vi "ClassPanel.vi"(8 "error in (no error)":errorcluster caption="entrée d'erreur (pas d'erreur)", 11 "ThorPM100A.lvclass":refnum<class "ThorPM100A.lvclass">) -> (0 "error out":errorcluster caption="sortie d'erreur", 3 "ThorPM100A.lvclass Out":refnum<class "ThorPM100A.lvclass">)   [LabVIEW 2019, in "ThorPM100A.lvclass"]
uses:
  ThorPM100A.lvclass
  C:/Programmes Labview/LabscanV1A/DevicesClass/BaseDevice/BaseDevice.lvclass
  ThorPM100A.lvclass/ThorPM100A.ctl
  BaseDevice/ClassQueueMess.ctl
  BaseDevice/BaseDevice.lvclass/BaseDevice.ctl
  BaseDevice/Accessor/GetBaseDataPath.vi
  BaseDevice/Accessor/GetClassEvent.vi
  <vilib>/Utility/error.llb/Error Cluster From Error Code.vi
  <vilib>/ErrorRing/Error Ring.xnode
panel:
  in  "TrigSourceRef":refnum<vi>
  out "ClearG":refnum<vi>
  in  "Clear":bool caption="MiseAJour"
  out "BaseDataPath":path
  out "VisaRes":refnum<visa-resource-name>
  out "AvgRef":refnum<vi>
  out "ViRef":refnum<vi>
  out "GraphRef":refnum<vi>
  out "DataRef":refnum<vi>
  out "GraphAct":bool
  in  "Graph":bool
  out "StartTime":dbl
  in  "PwIdx":i32
  out "PowerData":dbl[](array[numeric])
  out "Refresh count":u32=1 caption="Panel Refresh (s-1)" min=1 max=5 step=1
  in  "Panel Refresh":dbl=1.0 caption="Panel Refresh (s)" min=0.2 max=1000.0 step=0.2
  in  "Record":bool
  in  "Zero":bool
  in  "Conn/Dis":bool
  in  "Average":i16=60 caption="Average Cnt"
  in  "Attenuation":dbl=60.0 caption="Atten.(dB)" format="%^#.2e"
  in  "Range":dbl=60.0 caption="Range (W)" format="%^#.2e"
  in  "Autorange":bool
  in  "MainProgQ":refnum<queue>
  in  "MainProgQEvent":refnum<user-event>
  in  "Acq":bool
  in  "Stop":bool
  in  "Wavelength":dbl caption="Lambda(nm)" format="%.1f"
  in  "MiseAJour":bool
  out "Power":dbl=60.0 caption="Power (W)" min=0.1 step=0.1 format="%^#.3e"
  out "Init Program":bool
  # "PM100A PowerMeter"
  # "this MUST labeled with class name"
  # "this MUST be present and labeled \"Stop\" and \"Acq\""
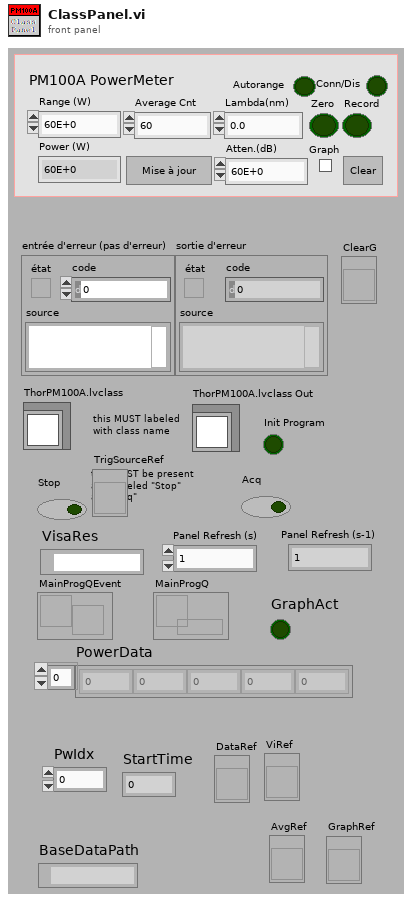
[diagram p1: front panel]
types:
  T1 = enum32{"Invalid", "Standard", "Closed", "Hidden", "Minimized", "Maximized"}
  T2 = cluster{"Max Val":dbl, "Curr.Val":dbl, "Meas.Avg":dbl, "Range":dbl}
  T3 = typedef "ClassQueueMess.ctl" = u16
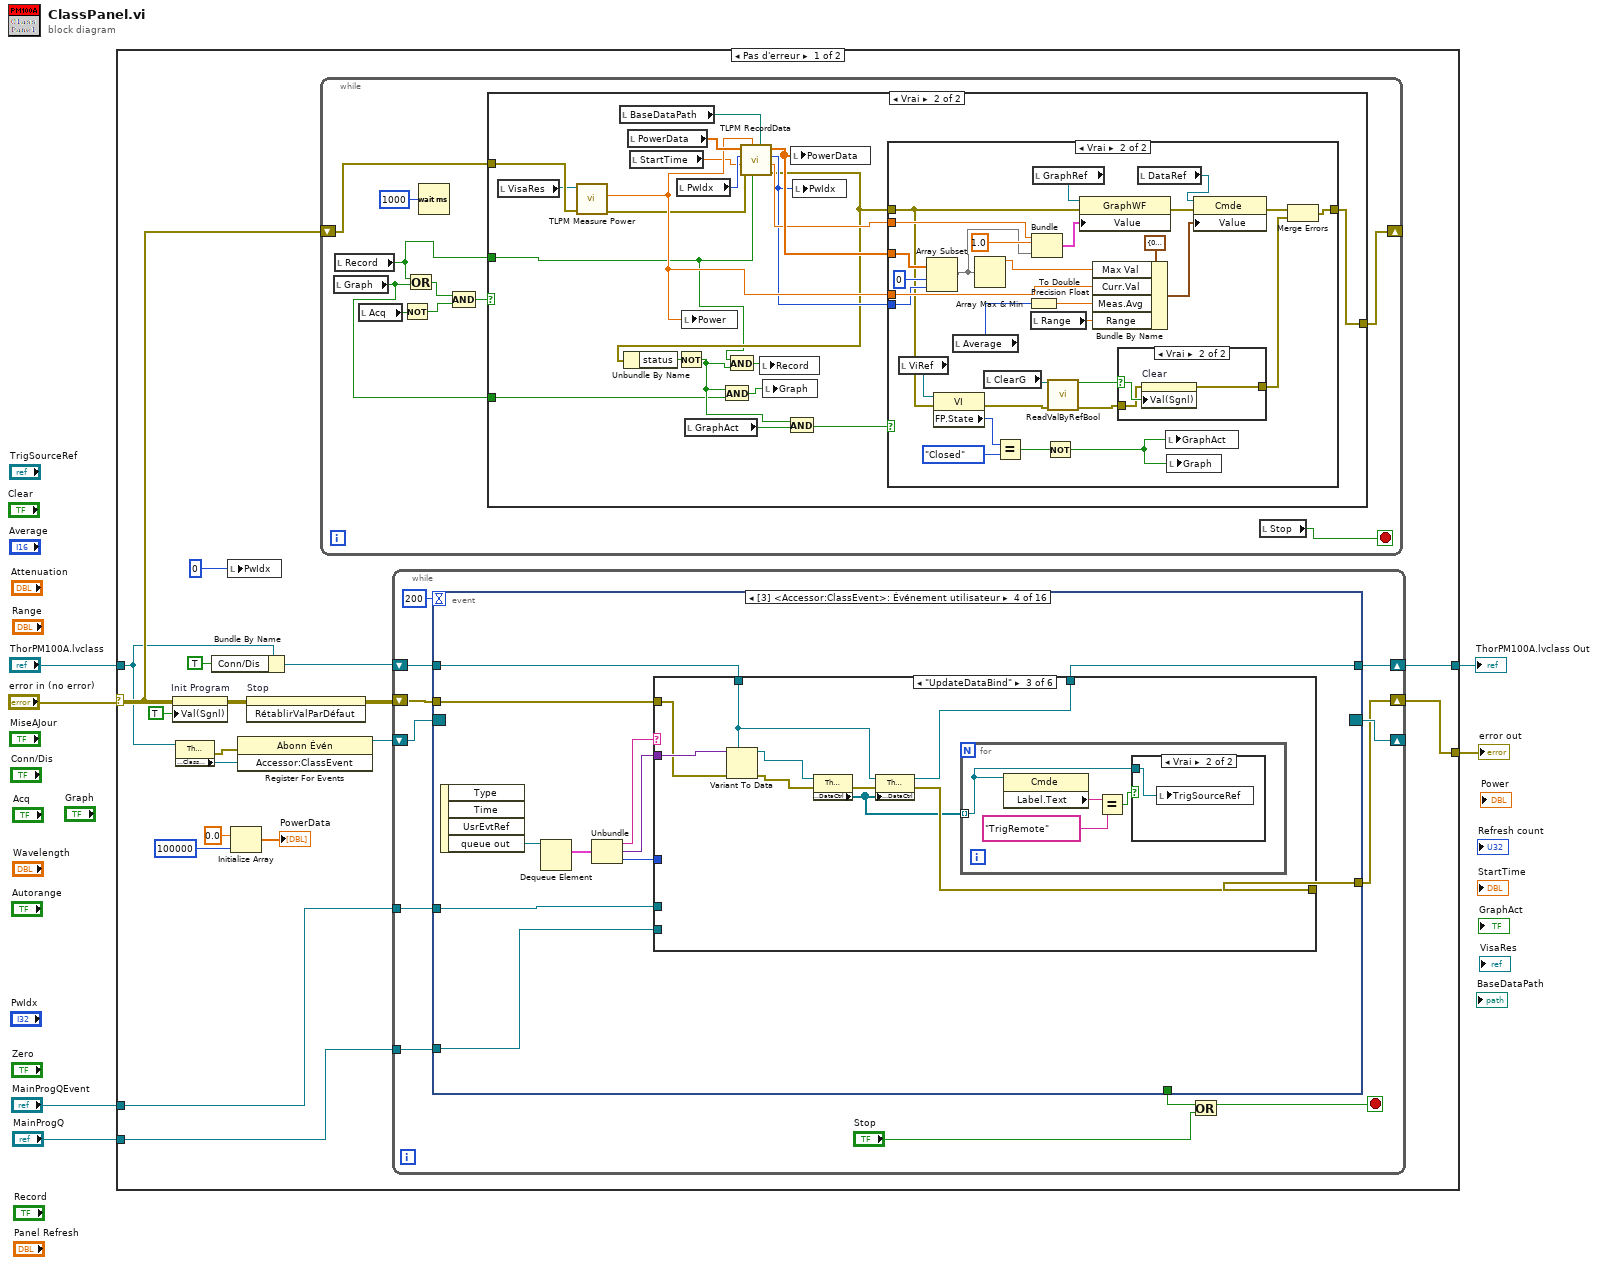
[diagram p0: block diagram]
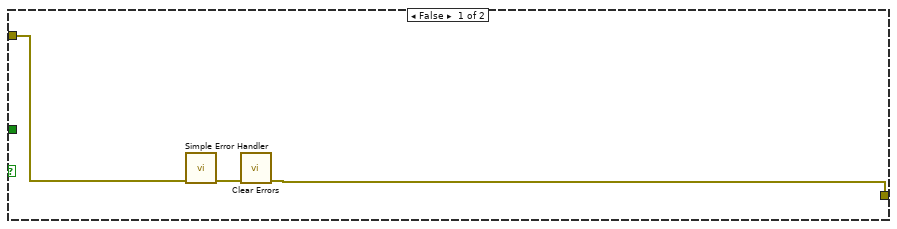
[diagram p2: hidden frame]
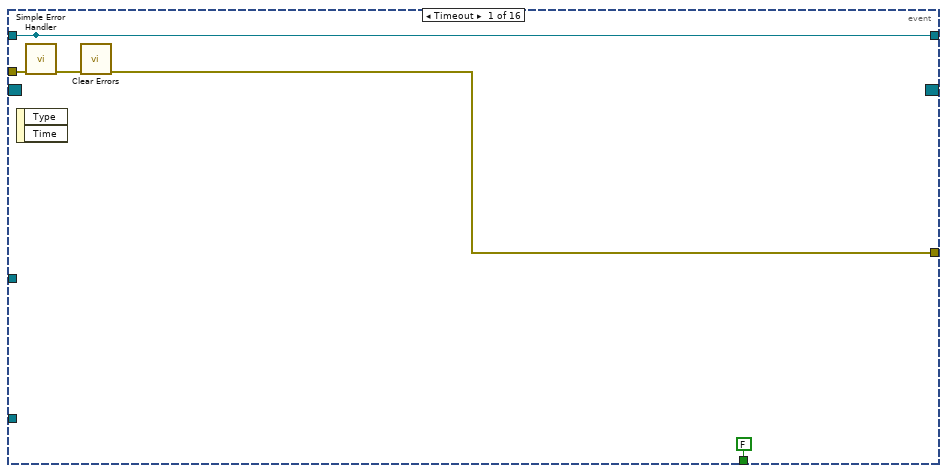
[diagram p5: hidden frame]
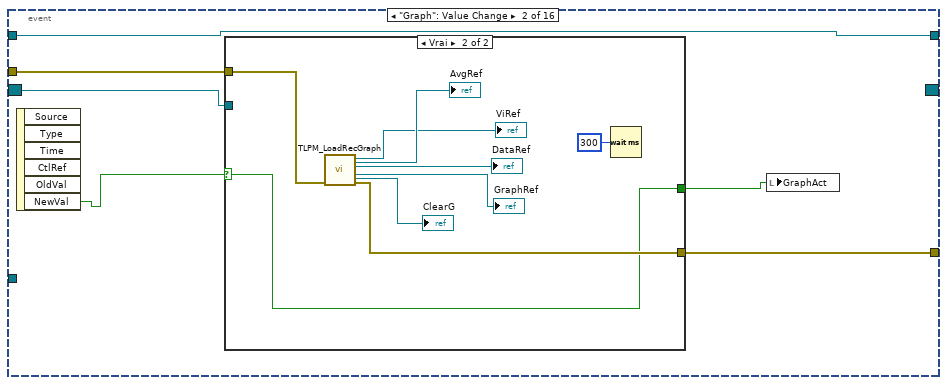
[diagram p6: hidden frame]
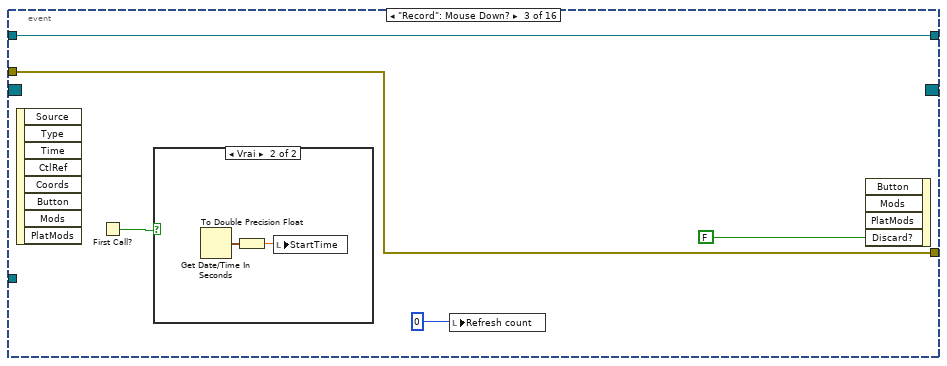
[diagram p8: hidden frame]
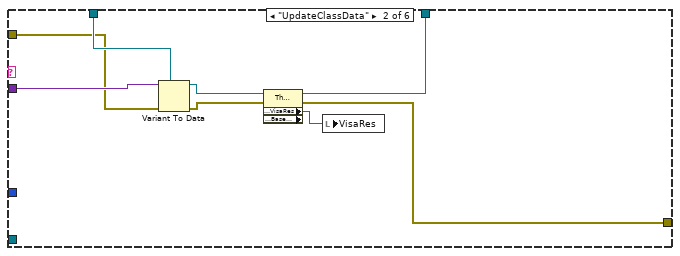
[diagram p11: hidden frame]
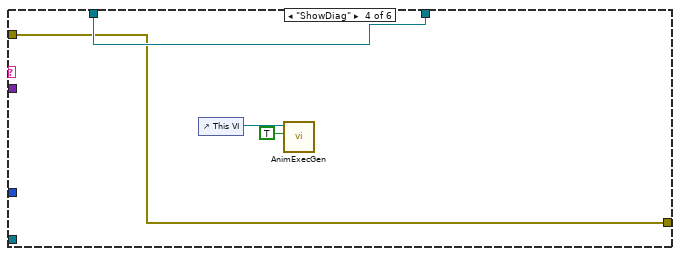
[diagram p13: hidden frame]
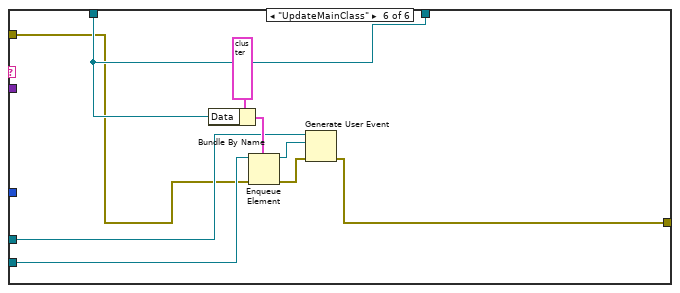
[diagram p15: hidden frame]
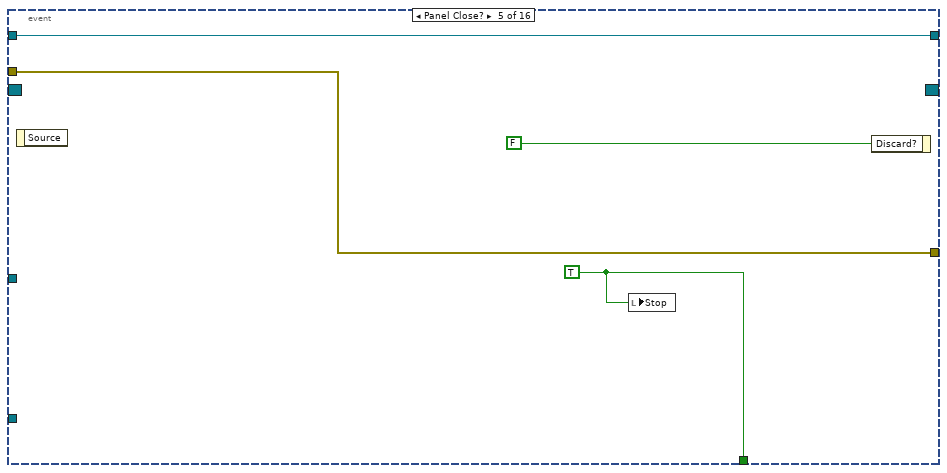
[diagram p16: hidden frame]
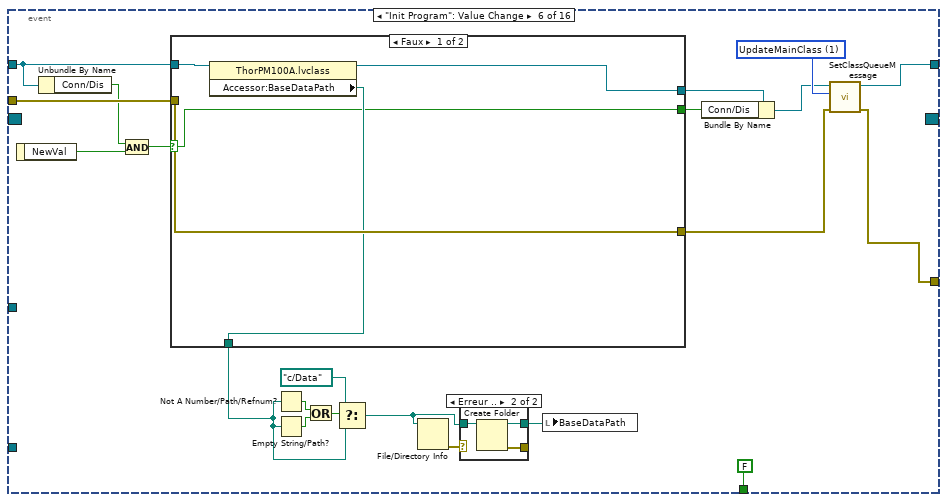
[diagram p17: hidden frame]
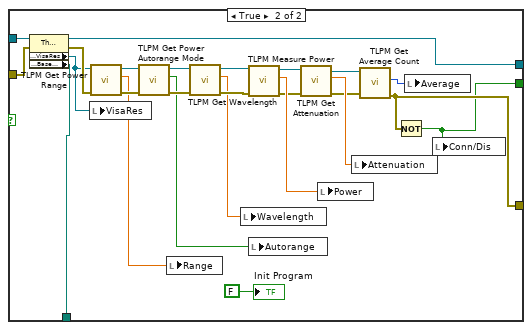
[diagram p19: hidden frame]
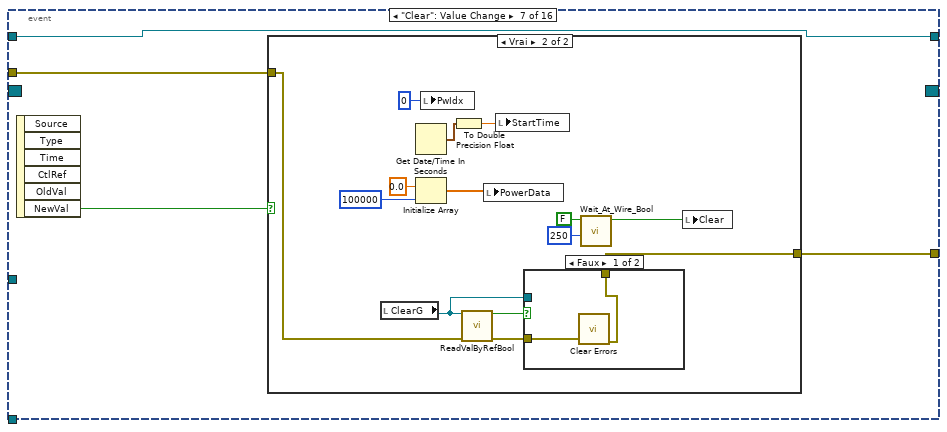
[diagram p20: hidden frame]
diagram:
  n1 = case shown="Pas d'erreur" "error in (no error)" {
    selector: "error in (no error)" -> [w10 w449]
    tunnel: [w24 w449] -> w5
    tunnel: "ThorPM100A.lvclass" -> [w9 w448]
    tunnel: [w22 w448] -> w3
    tunnel: "MainProgQEvent" -> [w16 _]
    tunnel: "MainProgQ" -> [w15 _]
    frame No Error {
      n2 = property on="Init Program" class="Bool (strict)"(error in=w10, "Val(Sgnl)"=TRUE ("Valeur (Signalisation)")) -> (error out=w21:errorcluster)  [unwired: 1 in, 1 out]
      n3 = property class="ThorPM100A.lvclass"(reference=w9) -> (error out=w19:errorcluster, "Accessor:ClassEvent"=w18:refnum<user-event>)  [unwired: 1 in, 1 out]
      n4 = Bundle By Name(cluster=w9, "Conn/Dis"=TRUE) -> (w7:refnum<class "ThorPM100A.lvclass">)
      n5 = local write "PwIdx"(u32 0 ("Power index")) -> ()
      n6 = Initialize Array(0.0 ("élément"), 100000 ("taille de la dimension")) -> (→"PowerData":dbl[])
      n7 = register-events(error in=w19, w18) -> (reference out=w17:refnum<event-registration>)  [unwired: 1 in, 1 out]
      n8 = invoke on="Stop" class="Bool (strict)" method="RétablirValParDéfaut"(error in=w21) -> (error out=w20:errorcluster)  [unwired: 2 in, 2 out]
      n9 = while {
        shift-right: [w28] -> _
        shift-left: w10 -> [w29]
        stop <- w32 stop-if-true
        n10 = local read "Graph"() -> (w25:bool)
        n11 = local read "Record"() -> (w26:bool)
        n12 = local read "Acq"() -> (w33:bool)
        n13 = Not(x=w33) -> (.not. x?=w34:bool)
        n14 = Or(x=w26, y=w25) -> (x .or. y?=w27:bool)
        n15 = Wait (ms)(milliseconds to wait=u32 1000 ("attente (ms)")) -> ()  [unwired: 1 out]
        n16 = Compound Arithmetic op=AND ("Opérateur arithmétique")(w27, w34) -> (w30:bool)
        n17 = case shown="Vrai" w30 {
          tunnel: [w35 w58] -> w28
          tunnel: w29 -> [w36 w49]
          tunnel: w26 -> [_ w41]
          tunnel: w25 -> [_ w38]
          frame False {
            n18 = call <vilib>:"Simple Error Handler.vi"("error in (no error)"=w36) -> ("error out"=w37:errorcluster)  [unwired: 4 in, 4 out]
            n19 = call <vilib>:"Clear Errors.vi"("error in (no error)"=w37) -> ("error out"=w35:errorcluster)  [unwired: 5 in, 1 out]
          }
          frame True {
            n20 = local read "VisaRes"() -> (w48:refnum<visa-resource-name>)
            n21 = call <instrlib>:"TLPM Measure Power.vi"("error in (no error)"=w49, "instrument handle"=w48) -> ("error out"=w45:errorcluster, "Power"=w53:dbl)  [unwired: 7 in, 1 out]
            n22 = local read "BaseDataPath"() -> (w46:path)
            n23 = local read "PowerData"() -> (w55:dbl[])
            n24 = local read "StartTime"() -> (w51:dbl)
            n25 = local read "PwIdx"() -> (w52:i32)
            n26 = local write "Power"(w53) -> ()
            n27 = local read "GraphAct"() -> (w56:bool)
            n28 = call "TLPM RecordData.vi"("BaseDataPath"=w46, "Save"=w41, "Power In"=w53, "error in (no error)"=w45, "StartTimeIn"=w51, "PwIdxIn"=w52, "PowerDataIn"=w55) -> ("error out"=w44:errorcluster, "StartTime"=w50:dbl, "PwIdxOut"=w47:i32, "PowerData"=w54:dbl[])  [unwired: 1 in]
            n29 = Unbundle By Name(w44) -> ("status"=w57:bool)
            n30 = Not(x=w57) -> (.not. x?=w40:bool)
            n31 = And(x=w40, y=w38) -> (x .and. y?=w39:bool)
            n32 = And(x=w41, y=w40) -> (x .and. y?=w42:bool)
            n33 = local write "Record"(w42) -> ()
            n34 = local write "Graph"(w39) -> ()
            n35 = And(x=w40, y=w56) -> (x .and. y?=w43:bool)
            n36 = local write "PowerData"(w54) -> ()
            n37 = local write "PwIdx"(w47) -> ()
            n38 = case shown="Vrai" w43 {
              tunnel: [w59 w64] -> w58
              tunnel: w44 -> [w59 w62]
              tunnel: w53 -> [_ w85]
              tunnel: w50 -> [_ w84]
              tunnel: w54 -> [_ w71]
              tunnel: w47 -> [_ w69]
              frame False {
              }
              frame True {
                n39 = local read "ViRef"() -> (w67:refnum<vi>)
                n40 = Array Subset(array=w71, index=0 ("indice"), length=w69) -> (w68:dbl[])
                n41 = property class="VI"(reference=w67, error in=w62) -> (error out=w61:errorcluster, "FP.State"=w81:T1)  [unwired: 1 out]
                n42 = local read "Average"() -> (w74:i16)
                n43 = Array Max & Min(array=w68) -> (max value=w75:dbl)  [unwired: 3 out]
                n44 = local read "ClearG"() -> (w60:refnum<vi>)
                n45 = Equal?(x=w81, y=T1."Closed") -> (x = y?=w79:bool)
                n46 = To Double Precision Float(number=w74) -> (double precision float=w73:dbl)
                n47 = local read "Range"() -> (w88:dbl)
                n48 = Bundle("StartTime"=w84, 1.0, w68) -> (w83:cluster{"StartTime":dbl, dbl, dbl[]})  [unwired: 1 in]
                n49 = local read "GraphRef"() -> (w82:refnum<vi>)
                n50 = Not(x=w79) -> (.not. x?=w78:bool)
                n51 = call <userlib>:"ReadValByRefBool.vi"("Control Ref"=w60, "error in"=w61) -> ("Valeur"=w66:bool, "error out"=w65:errorcluster)  [unwired: 12 in]
                n52 = property class="GraphWF"(reference=w82, error in=w62, "Value"=w83) -> (error out=w87:errorcluster)  [unwired: 1 out]
                n53 = Bundle By Name(cluster=T2 {"Max Val"=0.0, "Curr.Val"=0.0, "Meas.Avg"=0.0, "Range"=0.0} ("Data"), "Max Val"=w75, "Curr.Val"=w85, "Meas.Avg"=w73, "Range"=w88) -> (w76:T2)
                n54 = case shown="Vrai" w66 {
                  selector: w66 -> [_ w93]
                  tunnel: w65 -> [w90 w92]
                  tunnel: [w90 w91] -> w63
                  frame False {
                  }
                  frame True {
                    n55 = property on="Clear" class="Bool (strict)"(error in=w92, "Val(Sgnl)"=w93) -> (error out=w91:errorcluster)  [unwired: 1 in, 1 out]
                  }
                }
                n56 = local read "DataRef"() -> (w77:refnum<vi>)
                n57 = local write "GraphAct"(w78) -> ()
                n58 = local write "Graph"(w78) -> ()
                n59 = property class="Cmde"(reference=w77, error in=w87, "Value"=w76) -> (error out=w86:errorcluster)  [unwired: 1 out]
                n60 = Merge Errors(w86, w63) -> (w64:errorcluster)
              }
            }
          }
        }
        n61 = local read "Stop"() -> (w32:bool)
      }
      n62 = while {
        shift-right: [w94] -> w24
        shift-left: w20 -> [w104]
        shift-right: [w101] -> w22
        shift-left: w7 -> [w103]
        shift-right: [w97] -> _
        shift-left: w17 -> [w98]
        tunnel: w16 -> [w96]
        tunnel: w15 -> [w95]
        stop <- w100 stop-if-true
        n63 = event shown="[3] <Accessor:ClassEvent>: Événement utilisateur" {
          selector: w98 -> [_ w113 _ _ _ _ _ _ _ _ _ _ _ _ _ _]
          dyn-events: [_ _ _ _ _ _ _ _ _ _ _ _ _ _ _ _] -> w97
          timeout: 200 -> [_ _ _ _ _ _ _ _ _ _ _ _ _ _ _ _]
          tunnel: w104 -> [w109 w115 w131 w144 w187 w209 w245 w274 w312 w339 w389 w399 w409 w419 w427 w446]
          tunnel: [w106 w114 w131 w138 w187 w190 w246 w273 w311 w334 w386 w394 w405 w415 w423 w443] -> w94
          tunnel: w103 -> [w107 w111 w130 w145 w186 w207 w247 w271 w314 w340 w390 w400 w410 w420 w428 w447]
          tunnel: [FALSE _ _ _ w185 FALSE _ FALSE _ _ _ _ _ _ _ _] -> w102
          tunnel: [w107 w111 w130 w137 w186 w189 w247 w270 w313 w337 w385 w396 w408 w418 w426 w442] -> w101
          tunnel: w96 -> [_ _ _ w136 _ _ _ _ _ _ _ _ _ _ _ _]
          tunnel: w95 -> [_ _ _ w135 _ _ _ _ _ _ _ _ _ _ _ _]
          tunnel: [w107 _ _ _ _ _ _ _ _ _ _ _ _ _ _ _] -> _
          event Timeout {
            n64 = event-data() -> ()  [unwired: 1 in, 2 out]
            n65 = call <vilib>:"Simple Error Handler.vi"("error in (no error)"=w109) -> ("error out"=w108:errorcluster)  [unwired: 4 in, 4 out]
            n66 = call <vilib>:"Clear Errors.vi"("error in (no error)"=w108) -> ("error out"=w106:errorcluster)  [unwired: 5 in, 1 out]
          }
          event "Graph": Value Change {
            n67 = event-data() -> ("NewVal"=w116:bool)  [unwired: 1 in, 5 out]
            n68 = case shown="Vrai" w116 {
              selector: w116 -> [w117 w120]
              tunnel: w115 -> [w118 w127]
              tunnel: [w118 w122] -> w114
              tunnel: w113 -> [_ _]
              tunnel: [w117 w120] -> w112
              frame False {
              }
              frame True {
                n69 = call <instrlib>:"TLPM_LoadRecGraph.vi"("ErrIn(No Err)"=w127) -> ("ErrOut"=w122:errorcluster, "Graph"=→"GraphRef":refnum<vi>, "Data"=→"DataRef":refnum<vi>, "ViRef"=→"ViRef":refnum<vi>, "Clear"=→"ClearG":refnum<vi>, "Avg ref"=→"AvgRef":refnum<vi>)  [unwired: 5 in]
                n70 = Wait (ms)(milliseconds to wait=u32 300 ("attente (ms)")) -> ()  [unwired: 1 out]
              }
            }
            n71 = local write "GraphAct"(w112) -> ()
          }
          event "Record": Mouse Down? {
            n72 = event-data() -> ()  [unwired: 1 in, 8 out]
            n73 = First Call?() -> (First Call?: T/F=w129:bool)
            n74 = case shown="Vrai" w129 {
              frame False {
              }
              frame True {
                n75 = Get Date/Time In Seconds() -> (seconds since 1Jan1904=w134:timestamp)
                n76 = To Double Precision Float(number=w134) -> (double precision float=w133:dbl)
                n77 = local write "StartTime"(w133) -> ()
              }
            }
            n78 = local write "Refresh count"(u32 0 ("Refresh count")) -> ()
            n79 = event-data("Discard?"=FALSE ("Rejeter ?")) -> ()  [unwired: 4 in, 1 out]
          }
          event User Event {
            n80 = event-data() -> ("queue out"=w142:refnum<queue>)  [unwired: 1 in, 3 out]
            n81 = Dequeue Element(queue=w142) -> (element=w143:cluster{"Message":string, "Data":variant, i32})  [unwired: 2 in, 3 out]
            n82 = Unbundle(w143) -> ("Message"=w141:string, "Data"=w140:variant, w139:i32)
            n83 = case shown="\"UpdateDataBind\"" w141 {
              tunnel: w144 -> [w147 w151 w163 w170 w174 w177]
              tunnel: w140 -> [_ w155 w164 _ _ _]
              tunnel: w145 -> [w146 w154 w159 w171 w175 w180]
              tunnel: [w146 w152 w156 w171 w175 w180] -> w137
              tunnel: [w147 w149 w158 w170 w174 w176] -> w138
              tunnel: w139 -> [_ _ _ _ _ _]
              tunnel: w136 -> [_ _ _ _ _ w179]
              tunnel: w135 -> [_ _ _ _ _ w178]
              frame Default {
              }
              frame "UpdateClassData" {
                n84 = Variant To Data(error in=w151, type=w154, Variant=w155) -> (data=w153:refnum<class "ThorPM100A.lvclass">, error out=w150:errorcluster)
                n85 = property class="ThorPM100A.lvclass" props=["Accessor:VisaRes", "Accessor:BaseDataPath"](reference=w153, error in=w150) -> (reference out=w152:refnum<class "ThorPM100A.lvclass">, error out=w149:errorcluster, "Accessor:VisaRes"=w148:refnum<visa-resource-name>)  [unwired: 1 out]
                n86 = local write "VisaRes"(w148) -> ()
              }
              frame "UpdateDataBind" {
                n87 = Variant To Data(error in=w163, type=w159, Variant=w164) -> (data=w160:refnum<class "ThorPM100A.lvclass">, error out=w161:errorcluster)
                n88 = property class="ThorPM100A.lvclass"(reference=w160, error in=w161) -> (error out=w162:errorcluster, "Accessor:DataCtrl"=w157:refnum<vi>[])  [unwired: 1 out]
                n89 = property class="ThorPM100A.lvclass"(reference=w159, error in=w162, "Accessor:DataCtrl"=w157) -> (reference out=w156:refnum<class "ThorPM100A.lvclass">, error out=w158:errorcluster)
                n90 = for {
                  tunnel: w157 -> [w165] mode=indexing
                  n91 = property class="Cmde"(reference=w165) -> ("Label.Text"=w168:string)  [unwired: 1 in, 2 out]
                  n92 = Equal?(x=w168, y="TrigRemote") -> (x = y?=w166:bool)
                  n93 = case shown="Vrai" w166 {
                    tunnel: w165 -> [_ w169]
                    frame False {
                    }
                    frame True {
                      n94 = local write "TrigSourceRef"(w169) -> ()
                    }
                  }
                }
              }
              frame "ShowDiag" {
                n95 = control-ref of="This VI"() -> (w173:refnum<vi>)
                n96 = call <userlib>:"AnimExecGen.vi"("Animer l'exécution ?"=TRUE, "ViRef"=w173) -> ()  [unwired: 9 in, 1 out]
              }
              frame "MeasDone" {
              }
              frame "UpdateMainClass" {
                n97 = Bundle By Name(cluster=cluster{"Message":string, "Data":variant, i32} {"Message"="", "Data"=variant, 0} ("élément"), "Data"=w180) -> (w181:cluster{"Message":string, "Data":variant, i32})
                n98 = Enqueue Element(queue=w178, element=w181, error in (no error)=w177) -> (queue out=w184:refnum<queue>, error out=w183:errorcluster)  [unwired: 1 in, 1 out]
                n99 = Generate User Event(user event=w179, event data cluster=w184, error in=w183) -> (error out=w176:errorcluster)  [unwired: 1 in, 1 out]
              }
            }
          }
          event Panel Close? {
            w185 = TRUE
            n100 = event-data() -> ()  [unwired: 1 in, 1 out]
            n101 = local write "Stop"(w185) -> ()
            n102 = event-data("Discard?"=FALSE ("Rejeter ?")) -> ()  [unwired: 1 in, 1 out]
          }
          event "Init Program": Value Change {
            w193 = T3 1 items=["UpdateClassData", "UpdateMainClass", "UpdateDataBind", "ReInitDevice", "Custom", "ClosePan"] ("Menu déroulant")
            n103 = event-data() -> ("NewVal"=w204:bool)  [unwired: 1 in]
            n104 = Unbundle By Name(w207) -> ("Conn/Dis"=w205:bool)
            n105 = And(x=w205, y=w204) -> (x .and. y?=w206:bool)
            n106 = case shown="Faux" w206 {
              selector: w206 -> [w215 _]
              tunnel: w209 -> [w219 w241]
              tunnel: [w219 w225] -> w191
              tunnel: w207 -> [w218 w243]
              tunnel: [w217 w242] -> w195
              tunnel: [w216 w221] -> w196
              tunnel: [w215 w220] -> w194
              frame False {
                n107 = property class="ThorPM100A.lvclass"(reference=w218) -> (reference out=w217:refnum<class "ThorPM100A.lvclass">, "Accessor:BaseDataPath"=w216:path)  [unwired: 1 in, 1 out]
              }
              frame True {
                n108 = property class="ThorPM100A.lvclass"(reference=w243, error in=w241) -> (reference out=w242:refnum<class "ThorPM100A.lvclass">, error out=w240:errorcluster, "Accessor:VisaRes"=w222:refnum<visa-resource-name>, "Accessor:BaseDataPath"=w221:path)
                n109 = local write "VisaRes"(w222) -> ()
                n110 = call <instrlib>:"TLPM Get Power Range.vi"("error in (no error)"=w240, "instrument handle"=w222) -> ("error out"=w238:errorcluster, "Power Value"=w230:dbl, "instrument handle out"=w239:refnum<visa-resource-name>)  [unwired: 7 in]
                n111 = call <instrlib>:"TLPM Get Power Autorange Mode.vi"("error in (no error)"=w238, "instrument handle"=w239) -> ("error out"=w236:errorcluster, "Power Autorange Mode"=w235:bool, "instrument handle out"=w237:refnum<visa-resource-name>)  [unwired: 7 in]
                n112 = local write "Range"(w230) -> ()
                n113 = call <instrlib>:"TLPM Get Wavelength.vi"("error in (no error)"=w236, "instrument handle"=w237) -> ("error out"=w233:errorcluster, "Wavelength"=w232:dbl, "instrument handle out"=w234:refnum<visa-resource-name>)  [unwired: 7 in]
                n114 = local write "Wavelength"(w232) -> ()
                n115 = call <instrlib>:"TLPM Measure Power.vi"("error in (no error)"=w233, "instrument handle"=w234) -> ("error out"=w228:errorcluster, "Power"=w231:dbl, "instrument handle out"=w229:refnum<visa-resource-name>)  [unwired: 7 in]
                n116 = local write "Autorange"(w235) -> ()
                n117 = call <instrlib>:"TLPM Get Attenuation.vi"("error in (no error)"=w228, "instrument handle"=w229) -> ("error out"=w226:errorcluster, "Attenuation"=w227:dbl, "instrument handle out"=w224:refnum<visa-resource-name>)  [unwired: 7 in]
                n118 = local write "Power"(w231) -> ()
                n119 = local write "Attenuation"(w227) -> ()
                n120 = call <instrlib>:"TLPM Get Average Count.vi"("error in (no error)"=w226, "instrument handle"=w224) -> ("error out"=w225:errorcluster, "Average Count"=w223:i16)  [unwired: 7 in, 1 out]
                n121 = Not(x=w225) -> (.not. x?=w220:bool)
                n122 = local write "Average"(w223) -> ()
                n123 = local write "Conn/Dis"(w220) -> ()
                "Init Program" <- FALSE
              }
            }
            n124 = Not A Number/Path/Refnum?(number/path/refnum=w196) -> (NaN/Path/Refnum?=w202:bool)
            n125 = Empty String/Path?(string/path=w196) -> (empty?=w201:bool)
            n126 = Or(x=w202, y=w201) -> (x .or. y?=w200:bool)
            n127 = Select(t=path "c:/Data" ("cas vrai"), s=w200, f=w196) -> (s? t:f=w199:path)
            n128 = File/Directory Info(path=w199) -> (error out=w203:errorcluster)  [unwired: 1 in, 6 out]
            n129 = case shown="Erreur .." w203 {
              selector: w203 -> [w211 _]
              tunnel: w199 -> [w210 w214]
              tunnel: [w211 w213] -> _
              tunnel: [w210 w212] -> w198
              frame No Error {
              }
              frame Error {
                n130 = Create Folder(path (use dialog)=w214) -> (created path=w212:path, error out=w213:errorcluster)  [unwired: 2 in, 1 out]
              }
            }
            n131 = local write "BaseDataPath"(w198) -> ()
            n132 = Bundle By Name(cluster=w195, "Conn/Dis"=w194) -> (w192:refnum<class "ThorPM100A.lvclass">)
            n133 = call-dynamic "SetClassQueueMessage.vi"("ErrorIn(No Error)"=w191, "Menu déroulant"=w193, "DefaultDev.lvclass"=w192) -> ("sortie d'erreur"=w190:errorcluster, "DefaultDev.lvclass Out"=w189:refnum<class "ThorPM100A.lvclass">)  [unwired: 7 in]
          }
          event "Clear": Value Change {
            n134 = event-data() -> ("NewVal"=w248:bool)  [unwired: 1 in, 5 out]
            n135 = case shown="Vrai" w248 {
              tunnel: [w249 w251] -> w246
              tunnel: w245 -> [w249 w250]
              frame False {
              }
              frame True {
                n136 = local read "ClearG"() -> (w252:refnum<vi>)
                n137 = Get Date/Time In Seconds() -> (seconds since 1Jan1904=w256:timestamp)
                n138 = Initialize Array(0.0 ("élément"), 100000 ("taille de la dimension")) -> (w257:dbl[])
                n139 = local write "PwIdx"(0 ("PwIdx")) -> ()
                n140 = To Double Precision Float(number=w256) -> (double precision float=w255:dbl)
                n141 = call <userlib>:"ReadValByRefBool.vi"("Control Ref"=w252, "error in"=w250) -> ("Valeur"=w254:bool, "error out"=w253:errorcluster)  [unwired: 12 in]
                n142 = local write "PowerData"(w257) -> ()
                n143 = local write "StartTime"(w255) -> ()
                n144 = case shown="Faux" w254 {
                  tunnel: w253 -> [w265 w267]
                  tunnel: w252 -> [_ w269]
                  tunnel: [w264 w266] -> w251
                  frame False {
                    n145 = call <vilib>:"Clear Errors.vi"("error in (no error)"=w265) -> ("error out"=w264:errorcluster)  [unwired: 5 in, 1 out]
                  }
                  frame True {
                    n146 = call <userlib>:"WritebyWeakRefBool.vi"("error in"=w267, "Valeur"=FALSE, "Control Ref"=w269) -> ("error out"=w266:errorcluster)  [unwired: 8 in]
                  }
                }
                n147 = call <userlib>:"Wait_At_Wire_Bool.vi"("Wait (ms)"=u32 250, "error in (no error)"=FALSE) -> ("error out"=w263:bool)  [unwired: 7 in, 2 out]
                n148 = local write "Clear"(w263) -> ()
              }
            }
          }
          event "MiseAJour": Value Change {
            n149 = event-data() -> ("NewVal"=w275:bool)  [unwired: 1 in]
            n150 = case shown="Vrai" w275 {
              tunnel: w274 -> [w277 w302]
              tunnel: [w277 w280] -> w273
              tunnel: w271 -> [w276 w304]
              tunnel: [w276 w303] -> w270
              frame False {
              }
              frame True {
                n151 = property class="ThorPM100A.lvclass"(reference=w304, error in=w302) -> (reference out=w303:refnum<class "ThorPM100A.lvclass">, error out=w301:errorcluster, "Accessor:VisaRes"=w286:refnum<visa-resource-name>)
                n152 = call <instrlib>:"TLPM Get Power Range.vi"("error in (no error)"=w301, "instrument handle"=w286) -> ("error out"=w299:errorcluster, "Power Value"=w293:dbl, "instrument handle out"=w300:refnum<visa-resource-name>)  [unwired: 7 in]
                n153 = call <instrlib>:"TLPM Get Power Autorange Mode.vi"("error in (no error)"=w299, "instrument handle"=w300) -> ("error out"=w288:errorcluster, "Power Autorange Mode"=w298:bool, "instrument handle out"=w287:refnum<visa-resource-name>)  [unwired: 7 in]
                n154 = local write "Range"(w293) -> ()
                n155 = Wait (ms)(milliseconds to wait=u32 300 ("attente (ms)")) -> (millisecond timer value=w292:u32)
                n156 = call <instrlib>:"TLPM Get Wavelength.vi"("error in (no error)"=w288, "instrument handle"=w287) -> ()  [unwired: 7 in, 3 out]
                n157 = call <instrlib>:"TLPM Get Wavelength.vi"("error in (no error)"=w288, "instrument handle"=w287) -> ("error out"=w296:errorcluster, "Wavelength"=w295:dbl, "instrument handle out"=w297:refnum<visa-resource-name>)  [unwired: 7 in]
                n158 = flat-sequence {
                  tunnel: w292 -> [_]
                  frame #0 {
                    n159 = local write "MiseAJour"(FALSE ("MiseAJour")) -> ()
                  }
                }
                n160 = local write "Wavelength"(w295) -> ()
                n161 = call <instrlib>:"TLPM Measure Power.vi"("error in (no error)"=w296, "instrument handle"=w297) -> ("error out"=w290:errorcluster, "Power"=w294:dbl, "instrument handle out"=w289:refnum<visa-resource-name>)  [unwired: 7 in]
                n162 = local write "Autorange"(w298) -> ()
                n163 = local read "TrigSourceRef"() -> (w279:refnum<vi>)
                n164 = call <instrlib>:"TLPM Get Attenuation.vi"("error in (no error)"=w290, "instrument handle"=w289) -> ("error out"=w283:errorcluster, "Attenuation"=w285:dbl, "instrument handle out"=w282:refnum<visa-resource-name>)  [unwired: 7 in]
                n165 = local write "Attenuation"(w285) -> ()
                n166 = local write "Power"(w294) -> ()
                n167 = call <instrlib>:"TLPM Get Average Count.vi"("error in (no error)"=w283, "instrument handle"=w282) -> ("error out"=w281:errorcluster, "Average Count"=w284:i16)  [unwired: 7 in, 1 out]
                n168 = local write "Average"(w284) -> ()
                n169 = Not A Number/Path/Refnum?(number/path/refnum=w279) -> (NaN/Path/Refnum?=w278:bool)
                n170 = case shown="Faux" w278 {
                  tunnel: w281 -> [w308 w309]
                  tunnel: [w307 w309] -> w280
                  tunnel: w279 -> [w306 _]
                  frame False {
                    n171 = call <userlib>:"WritebyWeakRefBoolS.vi"("error in"=w308, "Valeur"=TRUE, "Control Ref"=w306) -> ("error out"=w307:errorcluster)  [unwired: 8 in]
                  }
                  frame True {
                  }
                }
              }
            }
          }
          event "Attenuation": Shortcut Menu Selection (User) {
            n172 = event-data() -> ("ItemTag"=w315:string)  [unwired: 1 in]
            n173 = case shown="\"Calc\"" w315 {
              tunnel: w314 -> [w317 w319]
              tunnel: [w317 w319] -> w313
              tunnel: w312 -> [w316 w318]
              tunnel: [w316 w322] -> w311
              frame Default {
              }
              frame "Calc" {
                n174 = call "Attenuation Calculator"("error in (no error)"=w318) -> ("Measured power (Watt)"=w320:dbl, "Reference power (Watt)"=w324:dbl, "OK"=w323:bool, "error out"=w321:errorcluster)  [unwired: 15 in]
                n175 = case shown="Vrai" w323 {
                  tunnel: w324 -> [_ w331]
                  tunnel: [w325 w326] -> w322
                  tunnel: w321 -> [w325 w327]
                  tunnel: w320 -> [_ w330]
                  frame False {
                  }
                  frame True {
                    n176 = Divide(x=w331, y=w330) -> (x/y=w329:dbl)
                    n177 = expression code="10*log(x)"(w329) -> (w328:dbl)
                    n178 = property on="Attenuation" class="NumNb (strict)"(error in=w327, "Val(Sgnl)"=w328) -> (error out=w326:errorcluster)  [unwired: 1 in, 1 out]
                  }
                }
              }
            }
          }
          event "Conn/Dis": Value Change {
            w336 = T3 1 items=["UpdateClassData", "UpdateMainClass", "UpdateDataBind", "ReInitDevice", "Custom", "ClosePan"] ("Menu déroulant")
            n179 = event-data() -> ("NewVal"=w341:bool)  [unwired: 1 in, 5 out]
            n180 = case shown="Vrai" w341 {
              tunnel: w340 -> [w346 w353]
              tunnel: [w346 w352] -> w338
              tunnel: [w344 w351] -> w335
              tunnel: w339 -> [w345 w350]
              tunnel: [w342 w347] -> w332
              frame False {
                w342 = FALSE ("Open")
                n181 = local read "VisaRes"() -> (w343:refnum<visa-resource-name>)
                n182 = call <instrlib>:"TLPM_OpenCloseConn.vi"("Open"=w342, "error in"=w345, "ConnID"=w343) -> ("error out"=w344:errorcluster)  [unwired: 7 in, 1 out]
              }
              frame True {
                n183 = call <instrlib>:"TLPM Find Resources.vi"("error in (no error)"=w350, "instrument handle"=refnum<visa-resource-name> refnum) -> ("error out"=w354:errorcluster, "Resource Count"=w356:u32)  [unwired: 7 in, 1 out]
                n184 = Greater Or Equal?(x=w356, y=u32 1) -> (x >= y?=w355:bool)
                n185 = case shown="Vrai" w355 {
                  tunnel: [w360 w382] -> w351
                  tunnel: w354 -> [_ w383]
                  tunnel: [_ w379] -> _
                  tunnel: [_ w370] -> w349
                  tunnel: w353 -> [w359 w372]
                  tunnel: [w359 w371] -> w352
                  frame False {
                    n186 = xnode "Menu déroulant d'erreurs"() -> ("sortie d'erreur"=w361:errorcluster)
                    n187 = call <vilib>:"Simple Error Handler.vi"("error in (no error)"=w361) -> ("error out"=w362:errorcluster)  [unwired: 4 in, 4 out]
                    n188 = call <vilib>:"Clear Errors.vi"("error in (no error)"=w362) -> ("error out"=w360:errorcluster)  [unwired: 5 in, 1 out]
                  }
                  frame True {
                    n189 = call <instrlib>:"TLPM Get Resource Name.vi"("error in (no error)"=w383, "Index (0)"=u32 0 ("Device Index")) -> ("error out"=w375:errorcluster, "Resource Name"=w377:string)  [unwired: 7 in, 1 out]
                    n190 = Type Cast(type=refnum<visa-resource-name> refnum ("VISA resource name"), x=w377) -> (*(type *) &x=w376:refnum<visa-resource-name>)
                    n191 = call <instrlib>:"TLPM_OpenCloseConn.vi"("Open"=TRUE, "error in"=w375, "Retry"=TRUE, "ConnID"=w376) -> ("error out"=w374:errorcluster, "connection ID"=w368:refnum<visa-resource-name>)  [unwired: 6 in]
                    n192 = property class="ThorPM100A.lvclass"(reference=w372, error in=w383, "Accessor:VisaRes"=w368) -> (reference out=w371:refnum<class "ThorPM100A.lvclass">)  [unwired: 1 out]
                    n193 = local write "VisaRes"(w368) -> ()
                    n194 = call <instrlib>:"TLPM Get Resource Information.vi"("error in (no error)"=w374, "instrument handle"=w368) -> ("error out"=w381:errorcluster, "Model Name"=w370:string, "Manufacturer"=w379:string)  [unwired: 4 in, 3 out]
                    n195 = call <vilib>:"Simple Error Handler.vi"("error in (no error)"=w381) -> ("error out"=w380:errorcluster)  [unwired: 4 in, 4 out]
                    n196 = call <vilib>:"Clear Errors.vi"("error in (no error)"=w380) -> ("error out"=w382:errorcluster)  [unwired: 5 in, 1 out]
                  }
                }
                n197 = Empty String/Path?(string/path=w349) -> (empty?=w348:bool)
                n198 = Not(x=w348) -> (.not. x?=w347:bool)
                n199 = local write "Conn/Dis"(w347) -> ()
              }
            }
            n200 = Bundle By Name(cluster=w338, "Conn/Dis"=w332) -> (w333:refnum<class "ThorPM100A.lvclass">)
            n201 = call-dynamic "SetClassQueueMessage.vi"("ErrorIn(No Error)"=w335, "Menu déroulant"=w336, "DefaultDev.lvclass"=w333) -> ("sortie d'erreur"=w334:errorcluster, "DefaultDev.lvclass Out"=w337:refnum<class "ThorPM100A.lvclass">)  [unwired: 7 in]
          }
          event "Wavelength": Value Change {
            n202 = event-data() -> ("NewVal"=w391:dbl)  [unwired: 1 in, 5 out]
            n203 = property class="ThorPM100A.lvclass"(reference=w390, error in=w389) -> (reference out=w385:refnum<class "ThorPM100A.lvclass">, error out=w387:errorcluster, "Accessor:VisaRes"=w388:refnum<visa-resource-name>)
            n204 = call <instrlib>:"TLPM Set Wavelength.vi"("error in (no error)"=w387, "Wavelength (0.0)"=w391, "instrument handle"=w388) -> ("error out"=w386:errorcluster)  [unwired: 7 in, 1 out]
          }
          event "Range": Value Change {
            n205 = event-data() -> ("NewVal"=w401:dbl)  [unwired: 1 in, 5 out]
            n206 = property class="ThorPM100A.lvclass"(reference=w400, error in=w399) -> (reference out=w396:refnum<class "ThorPM100A.lvclass">, error out=w397:errorcluster, "Accessor:VisaRes"=w398:refnum<visa-resource-name>)
            n207 = call <instrlib>:"TLPM Set Power Range.vi"("error in (no error)"=w397, "Power to Measure (0.0)"=w401, "instrument handle"=w398) -> ("error out"=w395:errorcluster, "instrument handle out"=w393:refnum<visa-resource-name>)  [unwired: 7 in]
            n208 = call <instrlib>:"TLPM Get Power Range.vi"("error in (no error)"=w395, "instrument handle"=w393) -> ("error out"=w394:errorcluster, "Power Value"=w392:dbl)  [unwired: 7 in, 1 out]
            n209 = local write "Range"(w392) -> ()
          }
          event "Attenuation": Value Change {
            n210 = event-data() -> ("NewVal"=w411:dbl)  [unwired: 1 in, 5 out]
            n211 = property class="ThorPM100A.lvclass"(reference=w410, error in=w409) -> (reference out=w408:refnum<class "ThorPM100A.lvclass">, error out=w402:errorcluster, "Accessor:VisaRes"=w403:refnum<visa-resource-name>)
            n212 = call <instrlib>:"TLPM Set Attenuation.vi"("error in (no error)"=w402, "Attenuation (0.0)"=w411, "instrument handle"=w403) -> ("error out"=w406:errorcluster, "instrument handle out"=w407:refnum<visa-resource-name>)  [unwired: 7 in]
            n213 = call <instrlib>:"TLPM Get Attenuation.vi"("error in (no error)"=w406, "instrument handle"=w407) -> ("error out"=w405:errorcluster, "Attenuation"=w404:dbl)  [unwired: 7 in, 1 out]
            n214 = local write "Attenuation"(w404) -> ()
          }
          event "Average": Value Change {
            n215 = event-data() -> ("NewVal"=w421:i16)  [unwired: 1 in, 5 out]
            n216 = property class="ThorPM100A.lvclass"(reference=w420, error in=w419) -> (reference out=w418:refnum<class "ThorPM100A.lvclass">, error out=w412:errorcluster, "Accessor:VisaRes"=w413:refnum<visa-resource-name>)
            n217 = call <instrlib>:"TLPM Set Average Count.vi"("error in (no error)"=w412, "Average Count (1)"=w421, "instrument handle"=w413) -> ("error out"=w416:errorcluster, "instrument handle out"=w417:refnum<visa-resource-name>)  [unwired: 7 in]
            n218 = call <instrlib>:"TLPM Get Average Count.vi"("error in (no error)"=w416, "instrument handle"=w417) -> ("error out"=w415:errorcluster, "Average Count"=w414:i16)  [unwired: 7 in, 1 out]
            n219 = local write "Average"(w414) -> ()
          }
          event "Zero": Value Change {
            n220 = event-data() -> ("NewVal"=w422:bool)  [unwired: 1 in, 5 out]
            n221 = property class="ThorPM100A.lvclass"(reference=w428, error in=w427) -> (reference out=w426:refnum<class "ThorPM100A.lvclass">, error out=w424:errorcluster, "Accessor:VisaRes"=w425:refnum<visa-resource-name>)
            n222 = case shown="Vrai" w422 {
              tunnel: w425 -> [_ w435]
              tunnel: w424 -> [w429 w434]
              tunnel: [w429 w431] -> w423
              frame False {
              }
              frame True {
                n223 = call <instrlib>:"TLPM Start Dark Offset Adjustment.vi"("error in (no error)"=w434, "instrument handle"=w435) -> ("error out"=w433:errorcluster)  [unwired: 8 in, 1 out]
                n224 = call <userlib>:"Wait_At_Wire_Err.vi"("Wait (ms)"=u32 250, "error in (no error)"=w433) -> ("error out"=w430:errorcluster)  [unwired: 7 in, 2 out]
                n225 = flat-sequence {
                  tunnel: [w437] -> w431
                  tunnel: w430 -> [w437]
                  frame #0 {
                    n226 = local write "Zero"(FALSE ("Zero")) -> ()
                  }
                }
              }
            }
          }
          event "Autorange": Value Change {
            w440 = u16 0 items=["ON"=1, "OFF"=0] ("Power Autorange Mode (ON)")
            w441 = u16 1 items=["ON"=1, "OFF"=0] ("Power Autorange Mode (ON)")
            n227 = event-data() -> ("NewVal"=w439:bool)  [unwired: 1 in]
            n228 = property class="ThorPM100A.lvclass"(reference=w447, error in=w446) -> (reference out=w442:refnum<class "ThorPM100A.lvclass">, error out=w444:errorcluster, "Accessor:VisaRes"=w445:refnum<visa-resource-name>)
            n229 = Select(t=w441, s=w439, f=w440) -> (s? t:f=w438:u16)
            n230 = call <instrlib>:"TLPM Set Power Autorange Mode.vi"("error in (no error)"=w444, "Power Autorange Mode (ON)"=w438, "instrument handle"=w445) -> ("error out"=w443:errorcluster)  [unwired: 7 in, 1 out]
          }
        }
        n231 = Or(x=w102, y="Stop") -> (x .or. y?=w100:bool)
      }
    }
    frame Error {
    }
  }
  "error out" <- w5
  "ThorPM100A.lvclass Out" <- w3
